vi "Varint Encoder uint64.vi"(9 "Array In":u8[](array[numeric]), 10 "Key":u32, 11 "Value":u64) -> (1 "Array":u8[](array[numeric]))   [LabVIEW 2021]
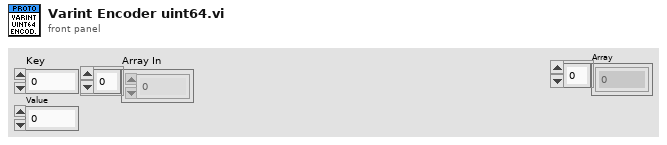
[diagram p1: front panel]
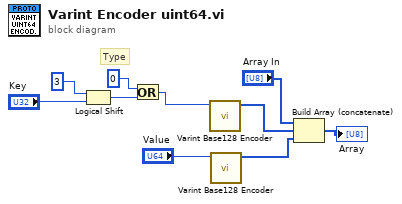
[diagram p0: block diagram]
diagram:
  # "Type"
  n1 = Logical Shift(y=i16 3, x="Key") -> (x << y=w8:u32)
  n2 = Or(x=u32 0, y=w8) -> (x .or. y?=w6:u32)
  n3 = call "Varint Base128 Encoder.vi"("Numeric"=w6) -> ("Array"=w4:u8[])  [unwired: 10 in]
  n4 = call "Varint Base128 Encoder.vi"("Numeric"="Value") -> ("Array"=w3:u8[])  [unwired: 10 in]
  n5 = Build Array (concatenate)("Array In", w4, w3) -> (→"Array":u8[])
